vi "FTW-File-FindLibrary.vi"(0 "Library File Pattern":path, 11 "error in":errorcluster) -> (6 "Library Filepath":path, 15 "error out":errorcluster)   [LabVIEW 2013]
panel:
  # "Inputs"
  # "Outputs"
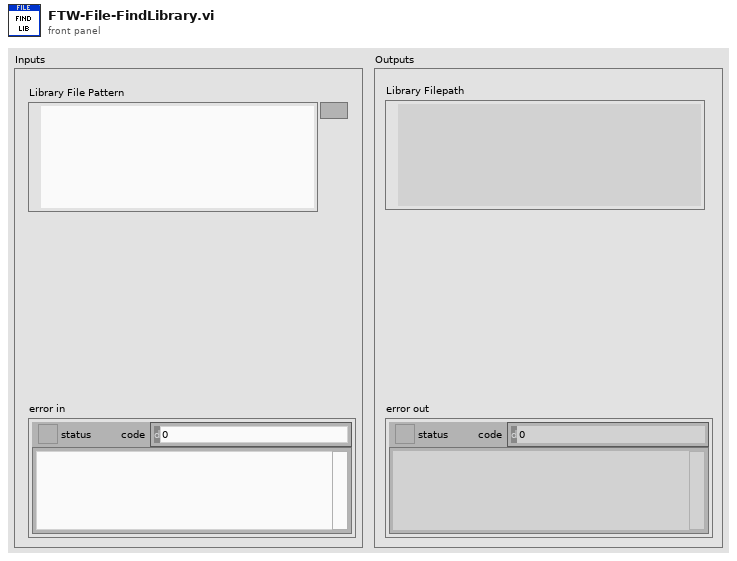
[diagram p1: front panel]
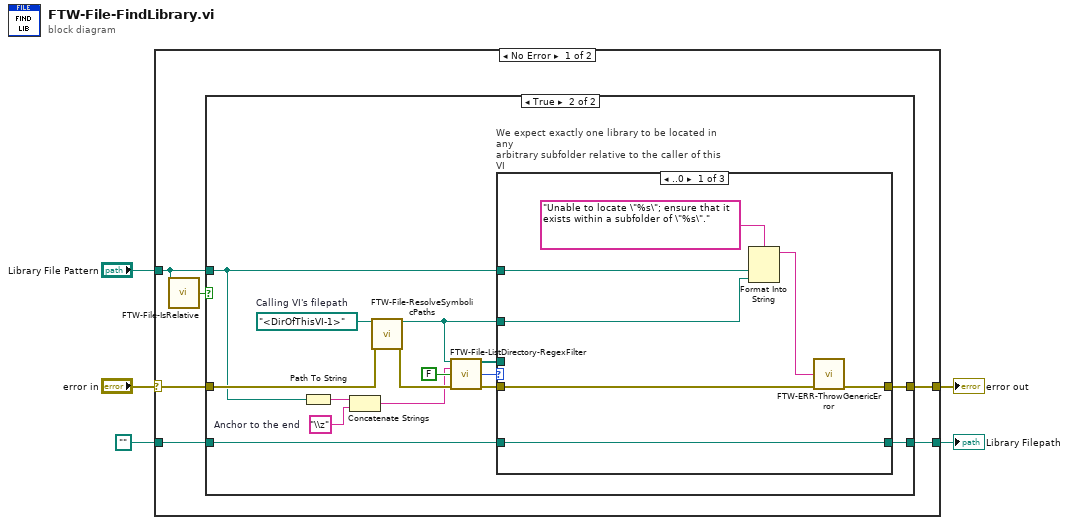
[diagram p0: block diagram]
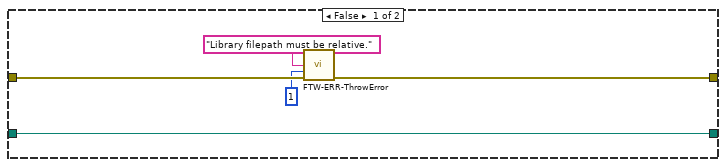
[diagram p2: hidden frame]
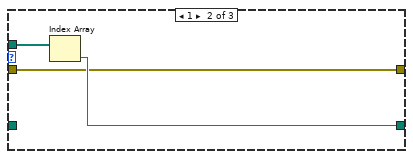
[diagram p3: hidden frame]
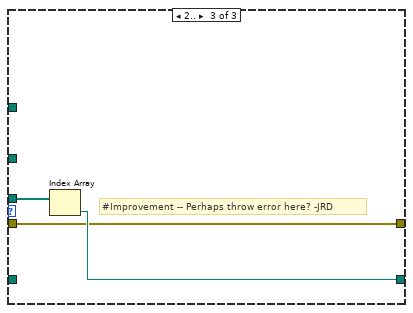
[diagram p4: hidden frame]
diagram:
  n1 = case shown="No Error" "error in" {
    selector: "error in" -> [w10 w46]
    tunnel: "Library File Pattern" -> [w7 _]
    tunnel: [w11 w46] -> w4
    tunnel: [w9 w45] -> w2
    tunnel: path "" -> [w8 w45]
    frame No Error {
      n2 = call "FTW-File-IsRelative.vi"("Filepath"=w7) -> ("Relative?"=w6:bool)
      n3 = case shown="True" w6 {
        tunnel: w10 -> [w16 w31]
        tunnel: [w15 w18] -> w11
        tunnel: w7 -> [_ w19]
        tunnel: [w12 w21] -> w9
        tunnel: w8 -> [w12 w20]
        frame False {
          n4 = call "FTW-ERR-ThrowError.vi"("Error Message"="Library filepath must be relative.", "Error Code"=1, "error in"=w16) -> ("error out"=w15:errorcluster)  [unwired: 12 in]
        }
        frame True {
          w23 = "\\z"  # Anchor to the end
          w28 = path "<DirOfThisVI-1>"  # Calling VI's filepath
          n5 = Path To String(path=w19) -> (string=w25:string)
          n6 = Concatenate Strings(w25, w23) -> (w24:string)
          n7 = call "FTW-File-ResolveSymbolicPaths.vi"("Unresolved Path"=w28, "error in"=w31) -> ("Resolved Path"=w17:path, "error out"=w29:errorcluster)  [unwired: 12 in]
          n8 = call "FTW-File-ListDirectory-RegexFilter.vi"("Directory to Search"=w17, "Filename Regex Filter"=w24, "Treat LLBs as Folders?"=FALSE, "error in"=w29) -> ("Matching Filepaths"=w22:path[], "Num Files Found"=w27:i32, "error out"=w26:errorcluster)  [unwired: 8 in, 1 out]
          n9 = case "We expect exactly one library to be located in any\narbitrary subfolder relative to the caller of this VI" shown="..0" w27 {
            tunnel: w26 -> [w32 w39 w42]
            tunnel: w22 -> [_ w41 w44]
            tunnel: [w38 w40 w43] -> w21
            tunnel: w20 -> [w38 _ _]
            tunnel: w19 -> [w37 _ _]
            tunnel: [w34 w39 w42] -> w18
            tunnel: w17 -> [w33 _ _]
            frame ..0 {
              n10 = Format Into String(format string="Unable to locate \"%s\"; ensure that it exists within a subfolder of \"%s\".", w37, w33) -> (resulting string=w35:string)  [unwired: 2 in, 1 out]
              n11 = call "FTW-ERR-ThrowGenericError.vi"("Error Message"=w35, "error in"=w32) -> ("error out"=w34:errorcluster)  [unwired: 13 in]
            }
            frame 1 {
              n12 = Index Array(array=w41) -> (element=w40:path)  [unwired: 1 in]
            }
            frame 2.. {
              # "#Improvement -- Perhaps throw error here? -JRD"
              n13 = Index Array(array=w44) -> (element=w43:path)  [unwired: 1 in]
            }
          }
        }
      }
    }
    frame Error {
    }
  }
  "error out" <- w4
  "Library Filepath" <- w2
